vi "GetChannelStatusTag.vi"(10 "channel id":string, 11 "tags":T1[](array[typedef])) -> (3 "channel status tag":T1)   [LabVIEW 2017, in "DeviceModelHelpers.lvlib"]
doc: "Returns a channel status tag based on the specified channel ID."
uses:
  <vilib>/addons/InsightCM/Utilities/DeviceModelHelpers/DeviceModelHelpers.lvlib
  <vilib>/addons/InsightCM/MessageBus/Base/controls/Tag.ctl
  <vilib>/addons/InsightCM/MessageBus/Base/controls/KeyValuePair.ctl
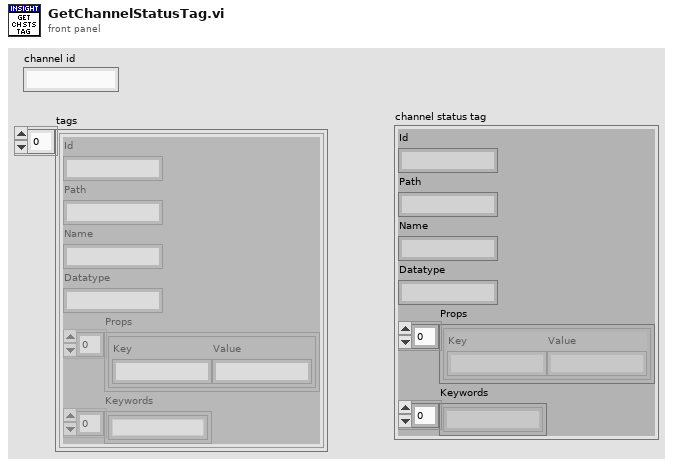
[diagram p1: front panel]
types:
  T1 = typedef "Tag.ctl" = cluster{"Id":string, "Path":string, "Name":string, "Datatype":string, "Props":T2[], "Keywords":string[]}
  T2 = typedef "KeyValuePair.ctl" = cluster{"Key":string, "Value":string}
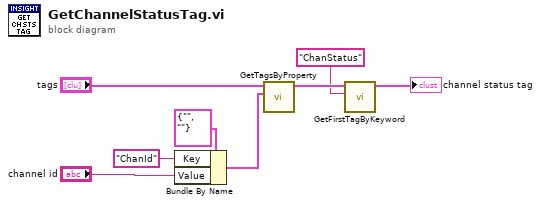
[diagram p0: block diagram]
diagram:
  n1 = Bundle By Name(cluster=T2 {"Key"="", "Value"=""} ("property"), "Key"="ChanId", "Value"="channel id") -> (w4:T2)
  n2 = call <vilib>:"GetTagsByProperty.vi"("property"=w4, "tags"="tags") -> ("matches"=w6:T1[])  [unwired: 9 in]
  n3 = call <vilib>:"GetFirstTagByKeyword.vi"("keyword"="ChanStatus", "tags"=w6) -> ("first tag"=→"channel status tag":T1)  [unwired: 9 in]
